vi "ExtendDevStatus_old.vi"(7 "error in":errorcluster, 9 "ON/OFF":bool, 10 "VISA resource name in":refnum<visa-resource-name>) -> (0 "error out":errorcluster, 2 "Extend Device Status":T1, 3 "VISA resource name out":refnum<visa-resource-name>)   [LabVIEW 2014]
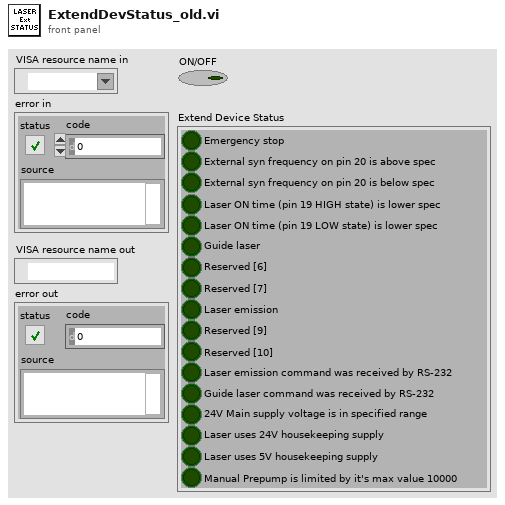
[diagram p1: front panel]
types:
  T1 = cluster{"Emergency stop":bool, "External syn frequency on pin 20 is above spec":bool, "External syn frequency on pin 20 is below spec":bool, "Laser ON time (pin 19 HIGH state) is lower spec":bool, "Laser ON time (pin 19 LOW state) is lower spec":bool, "Guide laser":bool, "Reserved [6]":bool, "Reserved [7]":bool, "Laser emission":bool, "Reserved [9]":bool, "Reserved [10]":bool, "Laser emission command was received by RS-232":bool, "Guide laser command was received by RS-232":bool, "24V Main supply voltage is in specified range":bool, "Laser uses 24V housekeeping supply":bool, "Laser uses 5V housekeeping supply":bool, "Manual Prepump is limited by it's max value 10000":bool}
  T2 = cluster{"Boolean array[0]":bool, "Boolean array[1]":bool, "Boolean array[2]":bool, "Boolean array[3]":bool, "Boolean array[4]":bool, "Boolean array[5]":bool, "Boolean array[6]":bool, "Boolean array[7]":bool, "Boolean array[8]":bool, "Boolean array[9]":bool, "Boolean array[10]":bool, "Boolean array[11]":bool, "Boolean array[12]":bool, "Boolean array[13]":bool, "Boolean array[14]":bool, "Boolean array[15]":bool, "Boolean array[16]":bool}
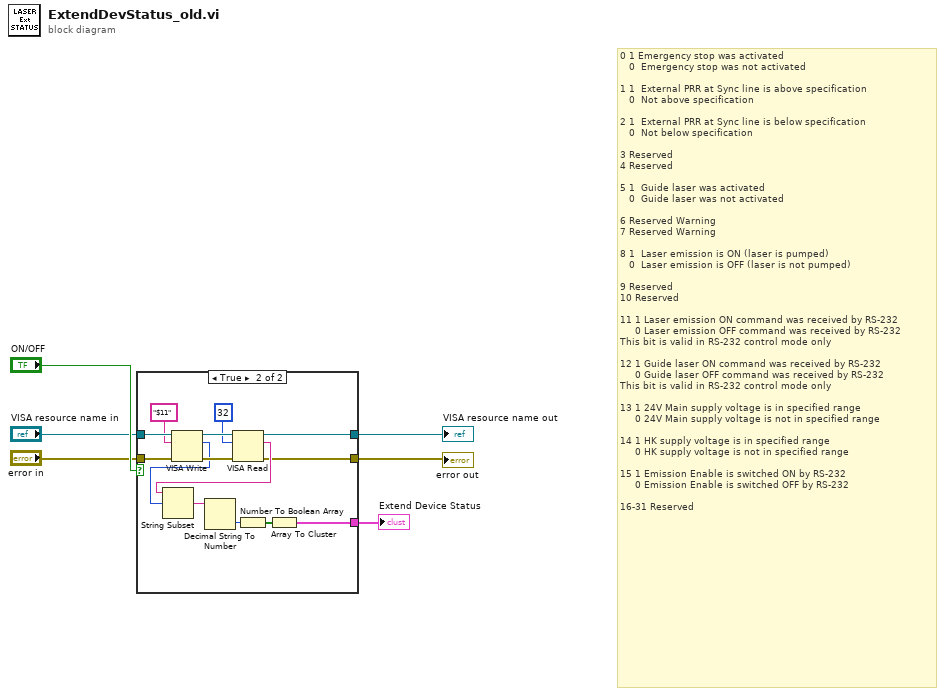
[diagram p0: block diagram]
diagram:
  # "0 1 Emergency stop was activated\n   0  Emergency stop was not activated\n\n1 1  External PRR at Sync line is above specification\n   0  Not above specification\n\n2 1  External PRR at Sync line is below specification\n   0  Not below specification\n\n3 Reserved\n4 Reserved\n\n5 1  Guide laser was activated\n   0  Guide laser was not activated\n\n6 Reserved Warning\n7 Reserved Warning\n\n8 1  Laser emission is ON (laser is pumped)\n   0  Laser emission is OFF (laser is not pumped) \n\n9 Reserved\n10 Reserved\n\n11 1 Laser emission ON command was received by RS-232\n     0 Laser emission OFF command was received by RS-232\nThis bit is valid in RS-232 control mode only\n\n12 1 Guide laser ON command was received by RS-232\n     0 Guide laser OFF command was received by RS-232\nThis bit is valid in RS-232 control mode only\n\n13 1 24V Main supply voltage is in specified range\n     0 24V Main supply voltage is not in specified range\n\n14 1 HK supply voltage is in specified range\n     0 HK supply voltage is not in specified range\n\n15 1 Emission Enable is switched ON by RS-232\n     0 Emission Enable is switched OFF by RS-232\n\n16-31 Reserved"
  n1 = case shown="True" "ON/OFF" {
    tunnel: "VISA resource name in" -> [w8 w20]
    tunnel: "error in" -> [w7 w19]
    tunnel: [w8 w10] -> w3
    tunnel: [w7 w9] -> w2
    tunnel: [_ w12] -> w1
    frame False {
    }
    frame True {
      n2 = VISA Write(VISA resource name=w20, write buffer="$11", error in (no error)=w19) -> (VISA resource name out=w21:refnum<visa-resource-name>, return count=w14:u32, error out=w22:errorcluster)
      n3 = VISA Read(VISA resource name=w21, byte count=u32 32, error in (no error)=w22) -> (VISA resource name out=w10:refnum<visa-resource-name>, read buffer=w15:string, error out=w9:errorcluster)  [unwired: 1 out]
      n4 = String Subset(string=w15, offset (0)=w14) -> (substring=w16:string)  [unwired: 1 in]
      n5 = Decimal String To Number(string=w16) -> (number=w17:i32)  [unwired: 2 in, 1 out]
      n6 = Number To Boolean Array(number=w17) -> (Boolean array=w13:bool[])
      n7 = Array To Cluster(array=w13) -> (cluster=w12:T2)
    }
  }
  "Extend Device Status" <- w1
  "VISA resource name out" <- w3
  "error out" <- w2
